vi "Off Wire Message to JSON.vi"(2 "error in":errorcluster, 3 "Off Wire Message":T1) -> (0 "error out":errorcluster, 1 "JSON string":string)   [LabVIEW 2016]
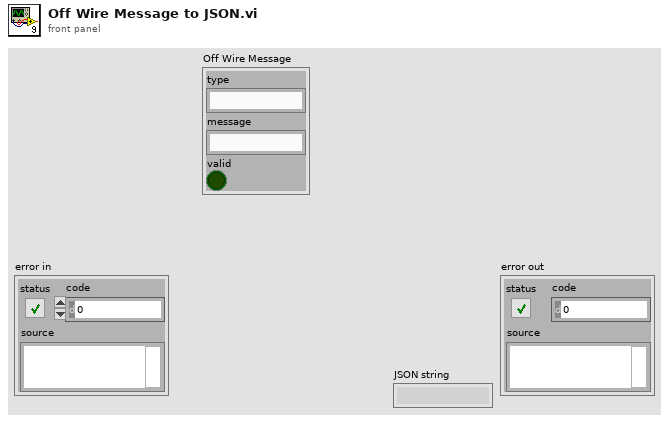
[diagram p1: front panel]
types:
  T1 = cluster{"type":string, "message":string, "valid":bool}
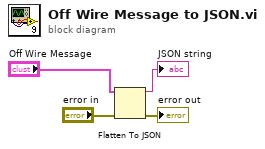
[diagram p0: block diagram]
diagram:
  n1 = Flatten To JSON(anything="Off Wire Message", error in (no error)="error in") -> (JSON string=→"JSON string":string, 11:→"error out":errorcluster)  [unwired: 1 in]
